vi "4.2 Arguments - Error As Arguments.vi"() -> ()   [LabVIEW 2017]
doc: "### 4.2 Arguments - Error As Arguments.vi\n\n#### Overview\n\nConverts a LabVIEW error cluster into a CSM-compatible error string, which allows the CSM core parse engine to process LabVIEW errors from the message queue. The converted error string uses the following format: `[Error: error-code] error-description-As-safe-argument-string`.\n\n#### Introduction\n\nThis example converts a LabVIEW error cluster into a CSM-compatible error string, which allows the CSM core parse engine to process LabVIEW errors from the message queue. The converted error string uses the following format: `[Error: error-code] error-description-As-safe-argument-string`. Furthermore, the CSM-Argument Type.vi gets the argument token, in this case `ErrStr`."
uses:
  user.lib/_NEVSTOP/Communicable State Machine(CSM)/AdvanceAPI/CSM - Revert Arguments-Safe String.vi
  user.lib/_NEVSTOP/Communicable State Machine(CSM)/AdvanceAPI/CSM - Make String Arguments Safe.vi
  user.lib/_NEVSTOP/Communicable State Machine(CSM)/AdvanceAPI/CSM - Keywords.vi
  user.lib/_NEVSTOP/Communicable State Machine(CSM)/_Shared/Trim Single-line Text.vi
  user.lib/_NEVSTOP/Communicable State Machine(CSM)/Communicable State Machine.lvlib
  user.lib/_NEVSTOP/Communicable State Machine(CSM)/_Shared/CSM Shared.lvlib
panel:
  out "argument token":string
  out "<ErrStr>[Error: 472]Error String 1%0AError String 2%0AError String 3":errorcluster
  out "[Error: 502]Error String 1%0AError String 2%0AError String 3":errorcluster
  out "Arguments":string
  out "error":errorcluster
  # "#CSM-Example Overview\n\nConverts a LabVIEW error cluster into a CSM-compatible error string, which allows the CSM core parse engine to process LabVIEW errors from the message queue. The converted error string uses the following format: `[Error: error-code] error-description-As-safe-argument-string`."
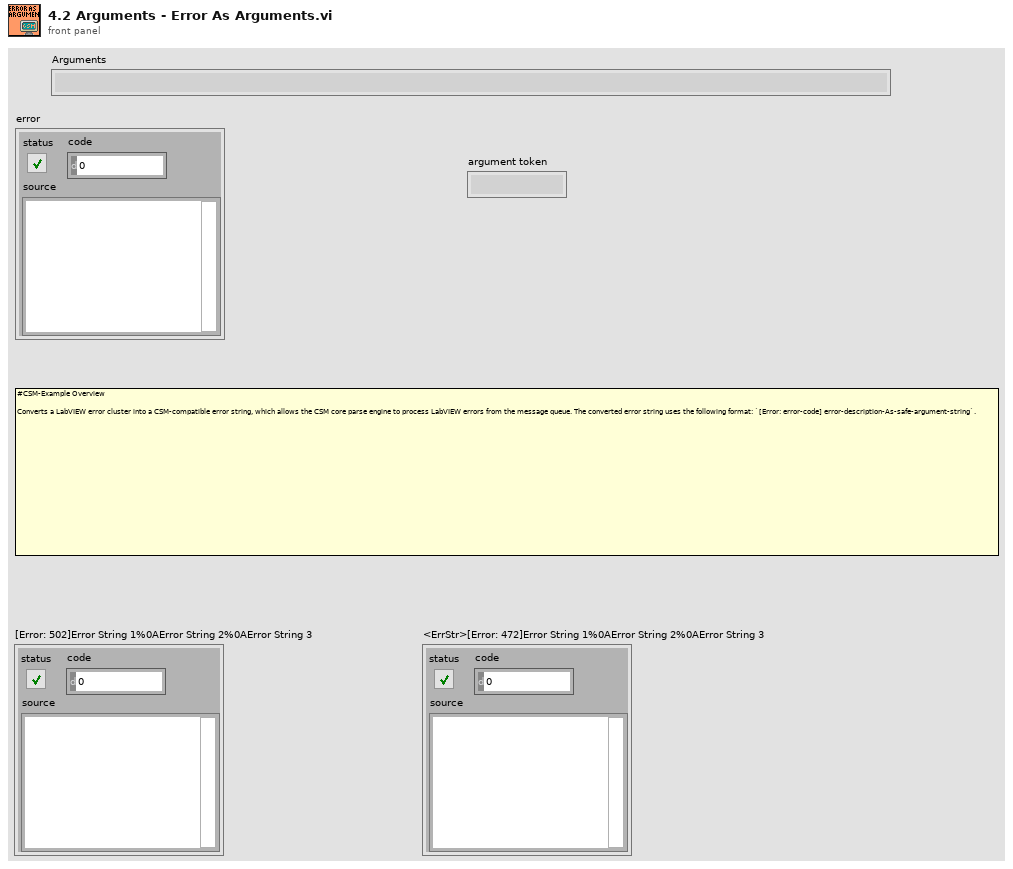
[diagram p1: front panel]
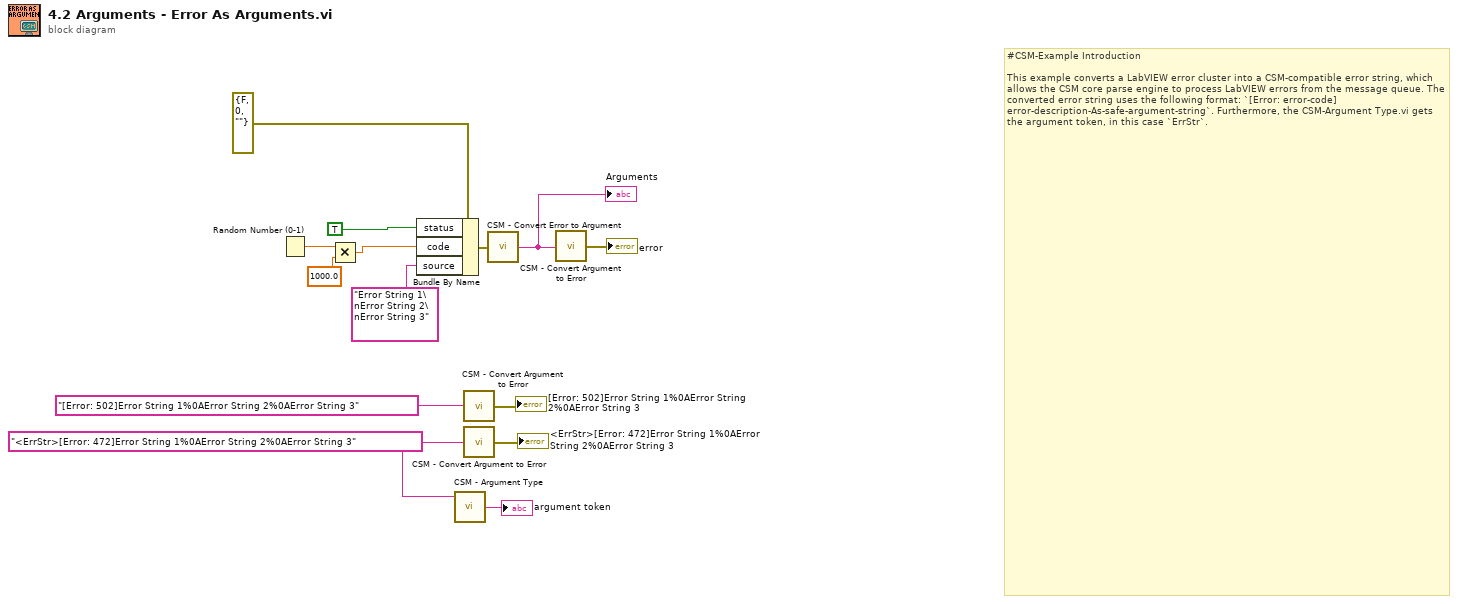
[diagram p0: block diagram]
diagram:
  w2 = "<ErrStr>[Error: 472]Error String 1%0AError String 2%0AError String 3" ("Arguments 2")
  # "#CSM-Example Introduction\n\nThis example converts a LabVIEW error cluster into a CSM-compatible error string, which allows the CSM core parse engine to process LabVIEW errors from the message queue. The converted error string uses the following format: `[Error: error-code] error-description-As-safe-argument-string`. Furthermore, the CSM-Argument Type.vi gets the argument token, in this case `ErrStr`."
  n1 = Random Number (0-1)() -> (number: 0 to 1=w9:dbl)
  n2 = Multiply(x=w9, y=1000.0) -> (x*y=w8:dbl)
  n3 = Bundle By Name(cluster=errorcluster {"status"=FALSE, "code"=0, "source"=""} ("error constant"), "status"=TRUE, "code"=w8, "source"="Error String 1\nError String 2\nError String 3") -> (w11:errorcluster)
  n4 = call "CSM - Argument Type.vi"("Arguments"=w2) -> ("Argument Type"=→"argument token":string)  [unwired: 3 in, 1 out]
  n5 = call "CSM - Convert Argument to Error.vi"("Argument"="[Error: 502]Error String 1%0AError String 2%0AError String 3" ("Arguments 2")) -> ("Error"=→"[Error: 502]Error String 1%0AError String 2%0AError String 3":errorcluster)  [unwired: 4 in]
  n6 = call "CSM - Convert Argument to Error.vi"("Argument"=w2) -> ("Error"=→"<ErrStr>[Error: 472]Error String 1%0AError String 2%0AError String 3":errorcluster)  [unwired: 4 in]
  n7 = call "CSM - Convert Error to Argument.vi"("Error"=w11) -> ("Argument"=w6:string)  [unwired: 4 in]
  "Arguments" <- w6
  n8 = call "CSM - Convert Argument to Error.vi"("Argument"=w6) -> ("Error"=→"error":errorcluster)  [unwired: 4 in]
